vi "Global Tube Measurement.vi"() -> ()   [LabVIEW 2019]
panel:
  in  "Tube Measurements":dbl[](array[numeric]) format="%.3f"
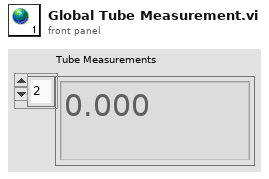
[diagram p1: front panel]
diagram:
